vi "GetAvailableCards.vi"(8 "error in (no error)":errorcluster, 11 "ClashRoyale in":refnum<class "StashRoyale.lvclass">) -> (0 "error out":errorcluster, 3 "ClashRoyale out":refnum<class "StashRoyale.lvclass">)   [LabVIEW 2020, in "StashRoyale.lvclass"]
uses:
  StashRoyale.lvclass
  StashRoyale.lvclass/StashRoyale.ctl
  ctl_ClientError.ctl
  ctl_AvailableCards.ctl
  ctl_Card.ctl
  <vilib>/httpClient/LabVIEWHTTPClient.lvlib
  <vilib>/addons/Tools/Unicode/UTF8 Tools.lvlib
  support/JSON.lvlibp
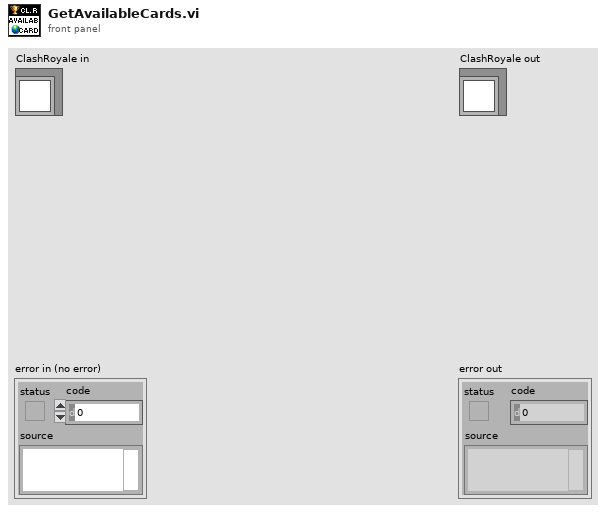
[diagram p1: front panel]
types:
  T1 = typedef "LabVIEWHTTPClient.lvlib/ClientHandle.ctl" = refnum<k1>
  T2 = typedef "StashRoyale.lvclass/ctl_ErrorCodes.ctl" = i32
  T3 = typedef "StashRoyale.lvclass/ctl_ClientError.ctl" = cluster{"reason":string, "message":string, "type":string}
  T4 = typedef "StashRoyale.lvclass/ctl_AvailableCards.ctl" = cluster{"items":T5[]}
  T5 = typedef "StashRoyale.lvclass/ctl_Card.ctl" = cluster{"name":string, "id":u32, "maxLevel":u8, "iconUrls":cluster{"medium":string}}
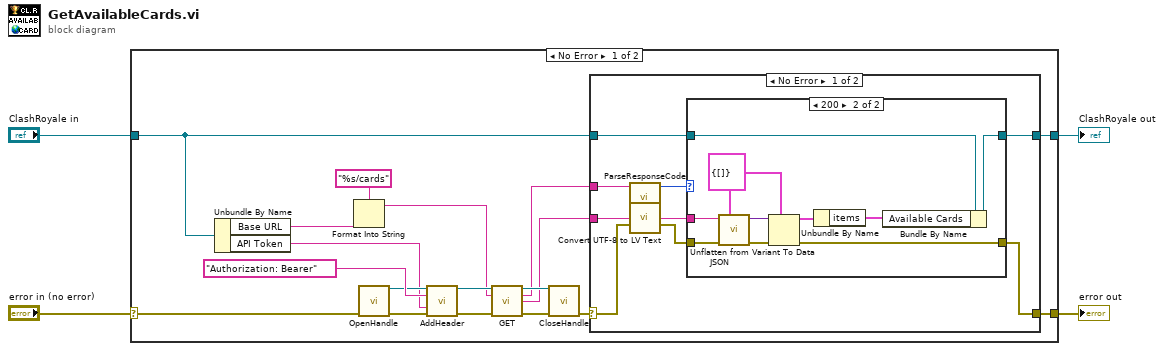
[diagram p0: block diagram]
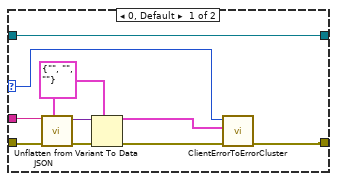
[diagram p2: hidden frame]
diagram:
  n1 = case shown="No Error" "error in (no error)" {
    selector: "error in (no error)" -> [w19 w55]
    tunnel: [w9 w55] -> w3
    tunnel: [w17 w54] -> w1
    tunnel: "ClashRoyale in" -> [w18 w54]
    frame No Error {
      n2 = Unbundle By Name(w18) -> ("Base URL"=w7:string, "API Token"=w10:string)
      n3 = Format Into String(format string="%s/cards" ("url"), w7) -> (resulting string=w5:string)  [unwired: 2 in, 1 out]
      n4 = call <vilib>:"OpenHandle.vi"("error in (no error)"=w19) -> ("client handle out"=w14:T1, "error out"=w11:errorcluster)  [unwired: 13 in]
      n5 = call <vilib>:"AddHeader.vi"("client handle"=w14, "header"="Authorization: Bearer", "value"=w10, "error in (no error)"=w11) -> ("client handle out"=w13:T1, "error out"=w12:errorcluster)  [unwired: 10 in]
      n6 = call <vilib>:"GET.vi"("client handle"=w13, "url"=w5, "error in (no error)"=w12) -> ("client handle out"=w22:T1, "headers"=w8:string, "body"=w20:string, "error out"=w21:errorcluster)  [unwired: 9 in]
      n7 = call <vilib>:"CloseHandle.vi"("client handle"=w22, "error in (no error)"=w21) -> ("error out"=w16:errorcluster)  [unwired: 13 in]
      n8 = case shown="No Error" w16 {
        selector: w16 -> [w28 w52]
        tunnel: w20 -> [w31 _]
        tunnel: w18 -> [w30 w53]
        tunnel: [w29 w53] -> w17
        tunnel: [w25 w52] -> w9
        tunnel: w8 -> [w24 _]
        frame No Error {
          n9 = call "ParseResponseCode.vi"("Response Header"=w24) -> ("response code (200)"=w23:T2)  [unwired: 10 in]
          n10 = call <vilib>:"Convert UTF-8 to LV Text.vi"("UTF-8 Text"=w31, "error in"=w28) -> ("LV Text"=w27:string, "error out"=w26:errorcluster)  [unwired: 12 in]
          n11 = case shown="200" w23 {
            selector: w23 -> [w33 _]
            tunnel: w30 -> [w41 w51]
            tunnel: [w41 w50] -> w29
            tunnel: w27 -> [w38 w46]
            tunnel: w26 -> [w37 w44]
            tunnel: [w32 w43] -> w25
            frame 0, Default {
              w36 = T3 {"reason"="", "message"="", "type"=""} ("ClientError")
              n12 = call "Unflatten from JSON.vi"("Type and Defaults"=w36, "error in (no error)"=w37, "JSON String"=w38) -> ("error out"=w39:errorcluster, "data"=w40:variant)  [unwired: 7 in]
              n13 = Variant To Data(error in=w39, type=w36, Variant=w40) -> (data=w34:T3, error out=w35:errorcluster)
              n14 = call "ClientErrorToErrorCluster.vi"("error in (no error)"=w35, "ClientError"=w34, "response code (200)"=w33) -> ("error out"=w32:errorcluster)  [unwired: 8 in]
            }
            frame 200 {
              w48 = T4 {"items"=[]} ("AvailableCards")
              n15 = call "Unflatten from JSON.vi"("Type and Defaults"=w48, "error in (no error)"=w44, "JSON String"=w46) -> ("error out"=w45:errorcluster, "data"=w49:variant)  [unwired: 7 in]
              n16 = Variant To Data(error in=w45, type=w48, Variant=w49) -> (data=w47:T4, error out=w43:errorcluster)
              n17 = Unbundle By Name(w47) -> ("items"=w42:T5[])
              n18 = Bundle By Name(cluster=w51, "Available Cards"=w42) -> (w50:refnum<class "StashRoyale.lvclass">)
            }
          }
        }
        frame Error {
        }
      }
    }
    frame Error {
    }
  }
  "error out" <- w3
  "ClashRoyale out" <- w1
